vi "Arm Position Check.vi"(1 "Threshold":dbl=5.0 format="%#_13g", 2 "Goal Angles (deg)":cluster{dbl, dbl, dbl}) -> (0 "Is Within Threshold":bool)   [LabVIEW 2020]
uses:
  GlobalArm.vi
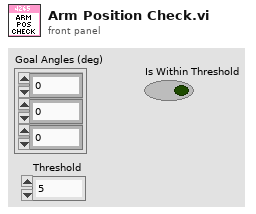
[diagram p1: front panel]
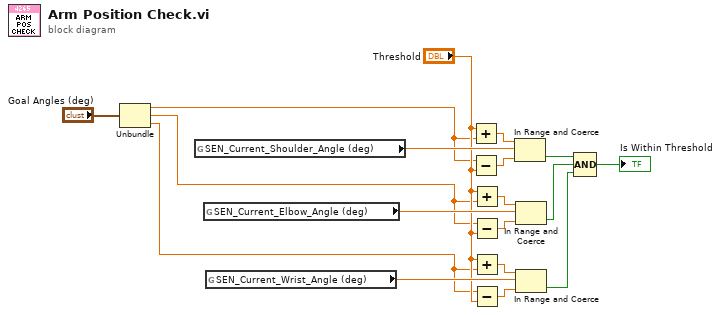
[diagram p0: block diagram]
diagram:
  n1 = Unbundle("Goal Angles (deg)") -> (w3:dbl, w2:dbl, w1:dbl)
  n2 = global read "GlobalArm.vi" "SEN_Current_Shoulder_Angle (deg)"() -> (w6:dbl)
  n3 = global read "GlobalArm.vi" "SEN_Current_Elbow_Angle (deg)"() -> (w9:dbl)
  n4 = global read "GlobalArm.vi" "SEN_Current_Wrist_Angle (deg)"() -> (w12:dbl)
  n5 = Add(x="Threshold", y=w3) -> (x+y=w8:dbl)
  n6 = Subtract(x=w3, y="Threshold") -> (x-y=w7:dbl)
  n7 = Add(x="Threshold", y=w2) -> (x+y=w10:dbl)
  n8 = Subtract(x=w2, y="Threshold") -> (x-y=w11:dbl)
  n9 = Add(x="Threshold", y=w1) -> (x+y=w13:dbl)
  n10 = Subtract(x=w1, y="Threshold") -> (x-y=w14:dbl)
  n11 = In Range and Coerce(upper limit=w8, x=w6, lower limit=w7) -> (In Range?=w15:bool)  [unwired: 1 out]
  n12 = In Range and Coerce(upper limit=w10, x=w9, lower limit=w11) -> (In Range?=w16:bool)  [unwired: 1 out]
  n13 = In Range and Coerce(upper limit=w13, x=w12, lower limit=w14) -> (In Range?=w17:bool)  [unwired: 1 out]
  n14 = Compound Arithmetic op=AND(w15, w16, w17) -> (→"Is Within Threshold":bool)
